vi "startUp.vi"(8 "error in (no error)":errorcluster, 10 "ScriptEvent":refnum<class "ScriptEvent.lvclass">, 11 "rfAction in":refnum<class "rfAction.lvclass">) -> (0 "error out":errorcluster, 3 "rfAction out":refnum<class "rfAction.lvclass">)   [LabVIEW 2011, in "Views.lvlib" / "ScriptEditor.lvlib" / "rfAction.lvclass"]
uses:
  rfAction.lvclass
  Tools/Scripting/ScriptingEvent/ScriptEvent.lvclass
  Tools/Scripting/ScriptingEvent/ScriptEvents/Rf Event/rf.lvclass
  rfAction.lvclass/rfAction.ctl
  ActionPanel.lvclass
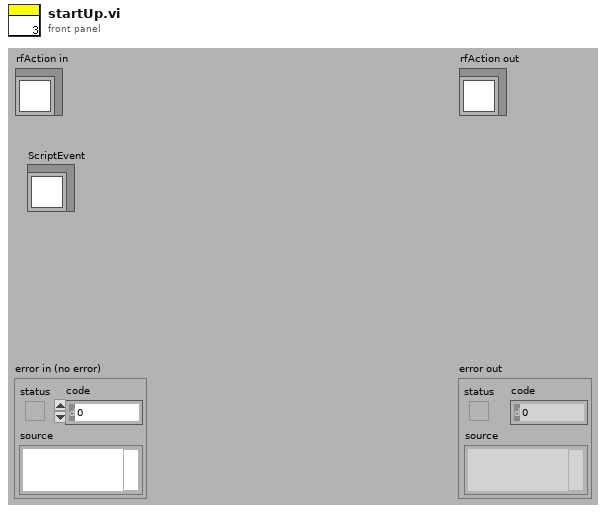
[diagram p1: front panel]
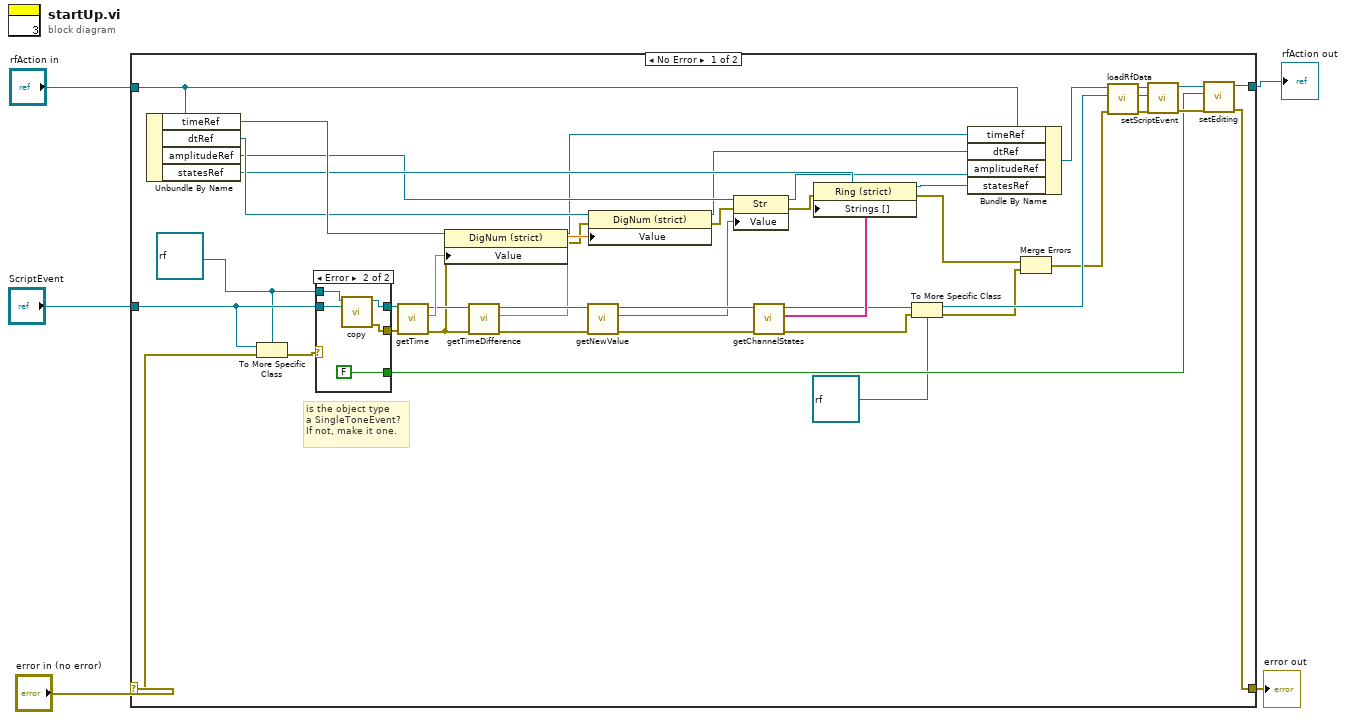
[diagram p0: block diagram]
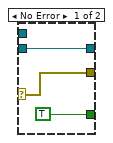
[diagram p2: hidden frame]
diagram:
  n1 = case shown="No Error" "error in (no error)" {
    selector: "error in (no error)" -> [w13 w59]
    tunnel: [w9 w59] -> w4
    tunnel: [w11 w58] -> w3
    tunnel: "rfAction in" -> [w26 w58]
    tunnel: "ScriptEvent" -> [w46 _]
    frame No Error {
      w7 = refnum<class "rf.lvclass"> refnum ("Tools.lvlib:Scripting.lvlib:rf.lvclass")
      # "is the object type\na SingleToneEvent?\nIf not, make it one."
      n2 = Unbundle By Name(w26) -> ("timeRef"=w45:refnum<vi>, "dtRef"=w44:refnum<vi>, "amplitudeRef"=w42:refnum<vi>, "statesRef"=w43:refnum<vi>)
      n3 = To More Specific Class(target class=w7, reference=w46, error in=w13) -> (error out=w49:errorcluster)  [unwired: 1 out]
      n4 = case shown="Error" w49 {
        selector: w49 -> [w51 _]
        tunnel: w46 -> [w52 w56]
        tunnel: w7 -> [_ w57]
        tunnel: [w51 w55] -> w48
        tunnel: [w52 w54] -> w47
        tunnel: [TRUE FALSE] -> w8
        frame No Error {
        }
        frame Error {
          n5 = call-dynamic "copy.vi"("ScriptEventForCopy"=w56, "rf in"=w57) -> ("error out"=w55:errorcluster, "rf out"=w54:refnum<class "rf.lvclass">)  [unwired: 8 in]
        }
      }
      n6 = call "getTime.vi"("error in (no error)"=w48, "ScriptEvent.lvclass in"=w47) -> ("error out"=w32:errorcluster, "time"=w41:dbl, "ScriptEvent.lvclass out"=w40:refnum<class "ScriptEvent.lvclass">)  [unwired: 7 in]
      n7 = property class="DigNum (strict)"(reference=w45, error in=w32, "Value"=w41) -> (reference out=w25:refnum<vi>, error out=w31:errorcluster)
      n8 = call "getTimeDifference.vi"("error in (no error)"=w32, "ScriptEvent.lvclass in"=w40) -> ("error out"=w33:errorcluster, "time difference"=w37:dbl, "ScriptEvent.lvclass out"=w39:refnum<class "ScriptEvent.lvclass">)  [unwired: 7 in]
      n9 = call "getNewValue.vi"("error in (no error)"=w33, "ScriptEvent.lvclass in"=w39) -> ("error out"=w34:errorcluster, "newValue"=w36:string, "ScriptEvent.lvclass out"=w38:refnum<class "ScriptEvent.lvclass">)  [unwired: 7 in]
      n10 = property class="DigNum (strict)"(reference=w44, error in=w31, "Value"=w37) -> (reference out=w24:refnum<vi>, error out=w30:errorcluster)
      n11 = property class="Str"(reference=w42, error in=w30, "Value"=w36) -> (reference out=w23:refnum<vi>, error out=w29:errorcluster)
      n12 = call-dynamic "getChannelStates.vi"("error in (no error)"=w34, "ScriptEvent in"=w38) -> ("error out"=w27:errorcluster, "statesValues"=w35:string[], "ScriptEvent out"=w28:refnum<class "ScriptEvent.lvclass">)  [unwired: 7 in]
      n13 = property class="Ring (strict)"(reference=w43, error in=w29, "Strings []"=w35) -> (reference out=w22:refnum<vi>, error out=w19:errorcluster)
      n14 = To More Specific Class(target class=refnum<class "rf.lvclass"> refnum ("Tools.lvlib:Scripting.lvlib:rf.lvclass"), reference=w28, error in=w27) -> (specific class reference=w20:refnum<class "rf.lvclass">, error out=w18:errorcluster)
      n15 = Bundle By Name(cluster=w26, "timeRef"=w25, "dtRef"=w24, "amplitudeRef"=w23, "statesRef"=w22) -> (w21:refnum<class "rfAction.lvclass">)
      n16 = Merge Errors(w19, w18) -> (w17:errorcluster)
      n17 = call "loadRfData.vi"("error in (no error)"=w17, "rf"=w20, "rfAction in"=w21) -> ("error out"=w15:errorcluster, "rf out"=w14:refnum<class "rf.lvclass">, "rfAction out"=w16:refnum<class "rfAction.lvclass">)  [unwired: 6 in]
      n18 = call "setScriptEvent.vi"("error in (no error)"=w15, "ScriptEvent.lvclass"=w14, "ActionPanel.lvclass in"=w16) -> ("error out"=w10:errorcluster, "ActionPanel.lvclass out"=w12:refnum<class "rfAction.lvclass">)  [unwired: 7 in]
      n19 = call "setEditing.vi"("error in (no error)"=w10, "editing?"=w8, "ActionPanel.lvclass in"=w12) -> ("error out"=w9:errorcluster, "ActionPanel.lvclass out"=w11:refnum<class "rfAction.lvclass">)  [unwired: 7 in]
    }
    frame Error {
    }
  }
  "error out" <- w4
  "rfAction out" <- w3
